vi "Get_IP_Number.vi"() -> (0 "bestAvailableName":string, 1 "IP Number":string)   [LabVIEW 2020]
panel:
  out "fresh?":bool
  in  "testArray":string[](array[string])=[""]
  out "scores":i32[](array[numeric])
  out "net address":u32[](array[numeric])
  out "Host Names":string[](array[string])
  out "IP Addresses":string[](array[string])
  in  "forceRefresh":bool
  # "Chooses the \"best\" available name for this machine from all assigned IPs, prioritising the lowest named, public, IP addresses"
  # "Default value of single empty element forces a listing of actual machine IPs\n\nType in values if required for testing"
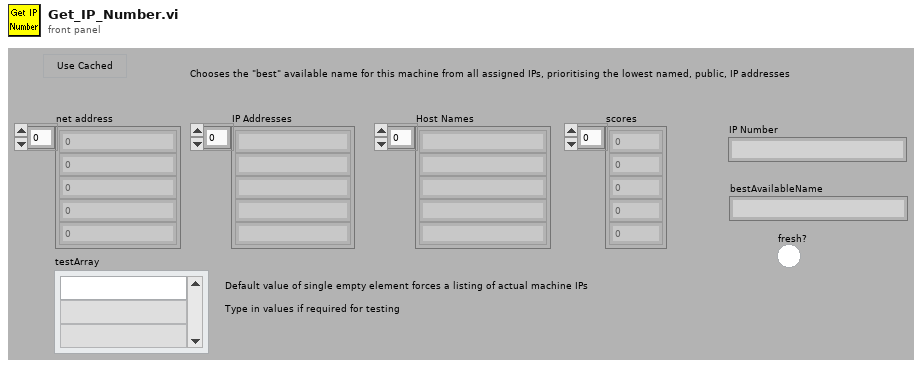
[diagram p1: front panel]
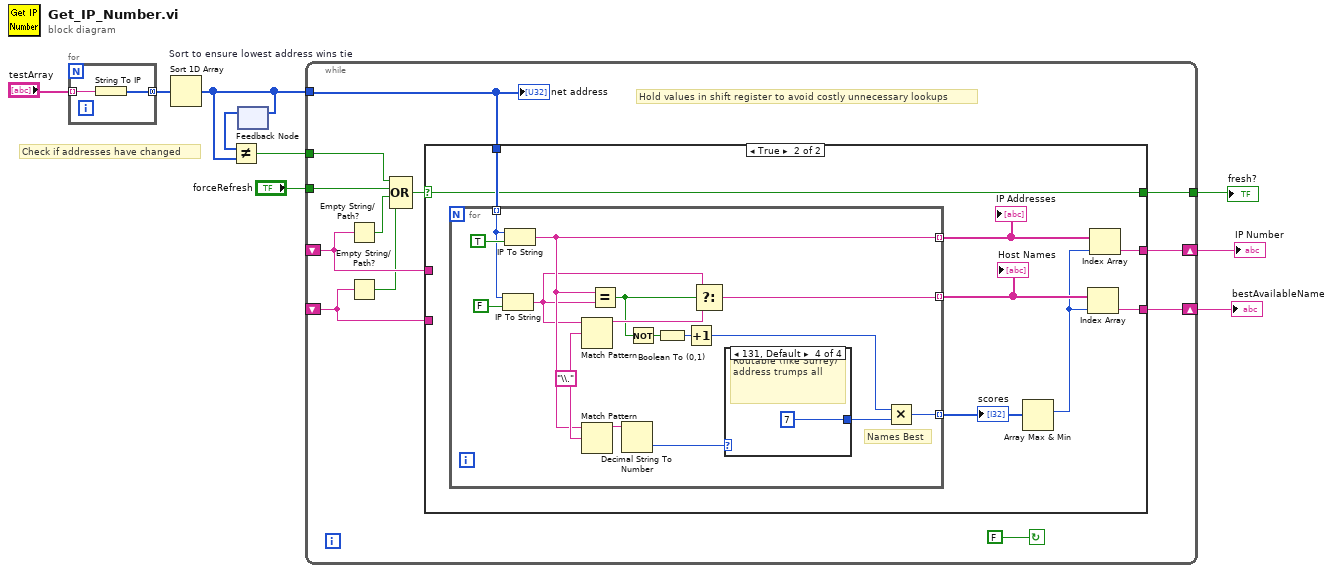
[diagram p0: block diagram]
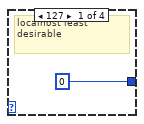
[diagram p3: hidden frame]
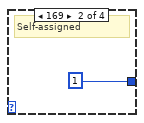
[diagram p4: hidden frame]
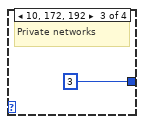
[diagram p5: hidden frame]
diagram:
  # "Check if addresses have changed"
  n1 = for {
    tunnel: [w11] -> w6 mode=concatenating
    tunnel: "testArray" -> [w10] mode=indexing
    n2 = String To IP(1:w10) -> (0:w11:u32[])
  }
  n3 = Sort 1D Array "Sort to ensure lowest address wins tie"(array=w6) -> (sorted array=w2:u32[])
  n4 = feedback #1() -> (w3:u32[])  [unwired: 1 in]
  n5 = Not Equal?(x=w3, y=w2) -> (x != y?=w4:bool)
  n6 = feedback-in #1(w2) -> ()
  n7 = while {
    shift-left: _ -> [w22]
    shift-right: [w23] -> w9
    shift-right: [w20] -> w8
    shift-left: _ -> [w17]
    tunnel: "forceRefresh" -> [w18]
    tunnel: w2 -> [w15]
    tunnel: w4 -> [w14]
    tunnel: [w12] -> w1
    stop <- FALSE continue-if-true
    # "Hold values in shift register to avoid costly unnecessary lookups"
    n8 = Empty String/Path?(string/path=w22) -> (empty?=w19:bool)
    n9 = Empty String/Path?(string/path=w17) -> (empty?=w16:bool)
    n10 = Compound Arithmetic op=OR(w14, w18, w19, w16) -> (w13:bool)
    n11 = case shown="True" w13 {
      selector: w13 -> [w24 w27]
      tunnel: [w26 w32] -> w23
      tunnel: w22 -> [w26 _]
      tunnel: [w25 w31] -> w20
      tunnel: w17 -> [w25 _]
      tunnel: w15 -> [_ w28]
      tunnel: [w24 w27] -> w12
      frame False {
        # "Don't look up if we have addresses, and nothing has changed"
      }
      frame True {
        n12 = for {
          tunnel: w28 -> [w48] mode=indexing
          tunnel: [w45] -> w33 mode=indexing
          tunnel: [w42] -> w34 mode=indexing
          tunnel: [w37] -> w30 mode=indexing
          w46 = "\\." ("regular expression")
          # "Names Best"
          n13 = IP To String(1:FALSE ("dot notation? (F)"), 2:w48) -> (0:w44:string)
          n14 = IP To String(1:TRUE ("dot notation? (F)"), 2:w48) -> (0:w45:string)
          n15 = Match Pattern(string=w44, regular expression=w46) -> (before substring=w43:string)  [unwired: 1 in, 3 out]
          n16 = Match Pattern(string=w45, regular expression=w46) -> (before substring=w47:string)  [unwired: 1 in, 3 out]
          n17 = Equal?(x=w45, y=w44) -> (x = y?=w41:bool)
          n18 = Decimal String To Number(string=w47) -> (number=w36:i32)  [unwired: 2 in, 1 out]
          n19 = Not(x=w41) -> (.not. x?=w40:bool)
          n20 = Boolean To (0,1)(Boolean=w40) -> (0, 1=w39:i16)
          n21 = Increment(x=w39) -> (x+1=w38:i16)
          n22 = Select(t=w44, s=w41, f=w43) -> (s? t:f=w42:string)
          n23 = case shown="131, Default" w36 {
            tunnel: [0 1 3 7] -> w35
            frame 127 {
              # "localhost least desirable"
            }
            frame 169 {
              # "Self-assigned"
            }
            frame 10, 172, 192 {
              # "Private networks"
            }
            frame 131, Default {
              # "Routable (like Surrey) address trumps all"
            }
          }
          n24 = Multiply(x=w38, y=w35) -> (x*y=w37:i32)
        }
        "IP Addresses" <- w33
        "Host Names" <- w34
        "scores" <- w30
        n25 = Array Max & Min(array=w30) -> (max index (indices)=w29:i32)  [unwired: 3 out]
        n26 = Index Array(array=w34, index=w29) -> (element=w31:string)
        n27 = Index Array(array=w33, index=w29) -> (element=w32:string)
      }
    }
    "net address" <- w15
  }
  "IP Number" <- w9
  "bestAvailableName" <- w8
  "fresh?" <- w1
